vi "CRYSet Plot Settings.vi"(4 "Fill To":i16, 6 "Style":u8, 7 "sAction":string, 8 "Color":u32, 9 "Row":i32, 10 "Legend Refnum":refnum<vi>, 11 "Type":enum16{"Curves", "Values", "Results", "WFM"}(ring)) -> ()   [LabVIEW 2013]
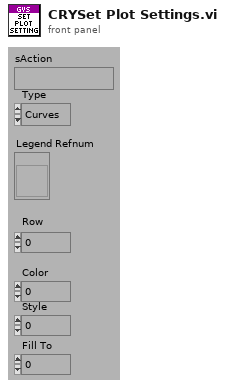
[diagram p1: front panel]
types:
  T1 = typedef "CRYData Cluster.ctl" = cluster{"Name":string, "Curve":cluster{"x":dbl, "y":dbl, "z":dbl}[], "X data":u16, "Y data":u16, "Z data":u16, "X axis":u16, "Y axis":u16, "Z axis":u16, "X unit":string, "Y unit":string, "Z unit":string, "X dB ref":dbl, "Y dB ref":dbl, "Z dB ref":dbl, "single val":bool, "protected":bool, "display X":bool, "display Y":bool, "display Z":bool, "Test Info":string, "Step No.":i32, "Plot Settings":cluster{"Color":u32, "Interpolation":u8, "Point Style":u8, "Line Style":u8, "Point Color":u32, "Line Width":u8, "Bar Plot Style":u8, "Fill To":i16}, "AutoProtect":bool}
  T2 = typedef "CRYWaveform Cluster.ctl" = cluster{"Waveform":cluster{"X0":dbl, "dX":dbl, "Y":sgl[]}, "X data":u16, "Y data":u16, "Y axis":u16, "X unit":string, "Y unit":string, "Y dB ref":dbl, "display Y":bool, "display X":bool, "Overload?":bool, "Test Info":string, "Step No.":i32, "Name":string, "protected":bool, "Sqc history":string[], "Signal Channel ID":i32, "Plot Settings":cluster{"Color":u32, "Interpolation":u8, "Point Style":u8, "Line Style":u8, "Point Color":u32, "Line Width":u8, "Bar Plot Style":u8, "Fill To":i16}, "AutoProtect":bool}
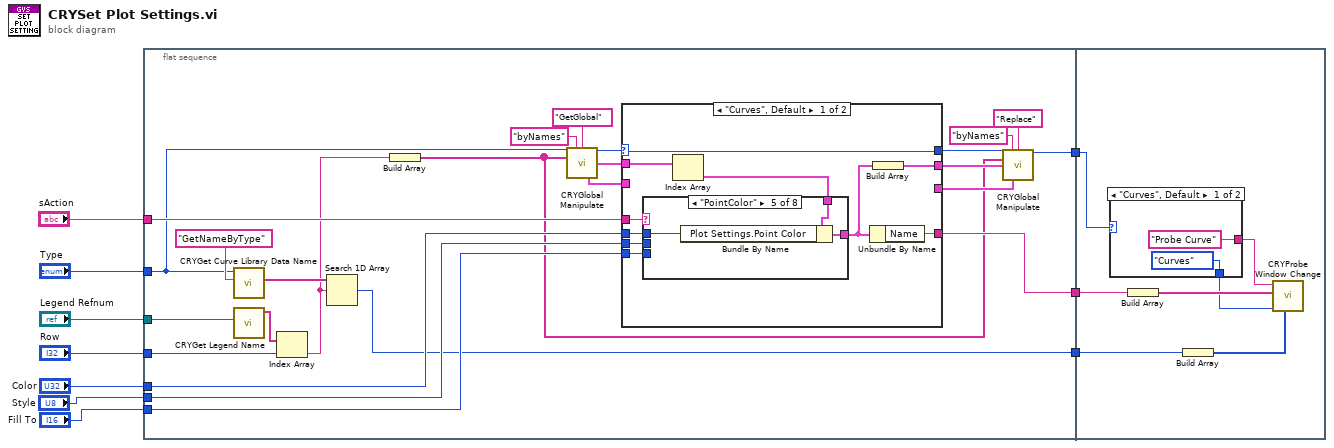
[diagram p0: block diagram]
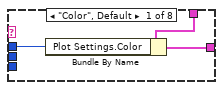
[diagram p2: hidden frame]
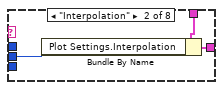
[diagram p3: hidden frame]
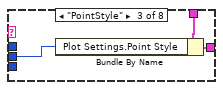
[diagram p4: hidden frame]
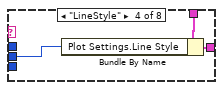
[diagram p5: hidden frame]
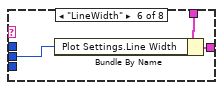
[diagram p6: hidden frame]
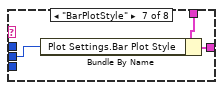
[diagram p7: hidden frame]
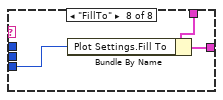
[diagram p8: hidden frame]
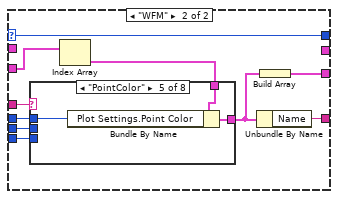
[diagram p9: hidden frame]
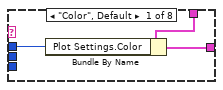
[diagram p10: hidden frame]
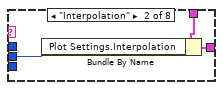
[diagram p11: hidden frame]
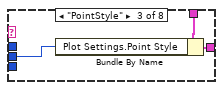
[diagram p12: hidden frame]
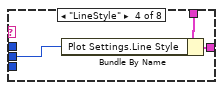
[diagram p13: hidden frame]
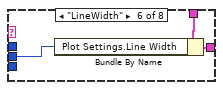
[diagram p14: hidden frame]
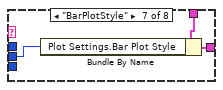
[diagram p15: hidden frame]
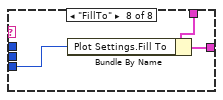
[diagram p16: hidden frame]
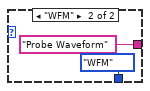
[diagram p17: hidden frame]
diagram:
  n1 = flat-sequence {
    tunnel: "Color" -> [w22]
    tunnel: "Legend Refnum" -> [w33]
    tunnel: "Row" -> [w32]
    tunnel: "Type" -> [w14]
    tunnel: [w18] -> w10
    tunnel: [w19] -> w9
    tunnel: "sAction" -> [w23]
    tunnel: "Style" -> [w21]
    tunnel: "Fill To" -> [w20]
    tunnel: [w17] -> w1
    tunnel: w10 -> [w109]
    tunnel: w9 -> [w106]
    tunnel: w1 -> [w104]
    frame #0 {
      n2 = call "CRYGet Curve Library Data Name.vi"("sAction"="GetNameByType", "Type"=w14) -> ("sNames"=w35:string[])  [unwired: 4 in, 5 out]
      n3 = call "CRYGet Legend Name.vi"("MCListbox Refnum"=w33) -> ("Names Out"=w34:string[])  [unwired: 1 in, 9 out]
      n4 = Index Array(array=w34, index=w32) -> (element=w13:string)
      n5 = Search 1D Array(1D array=w35, element=w13) -> (index of element=w19:i32)  [unwired: 1 in]
      n6 = Build Array(w13) -> (w12:string[])
      n7 = call "CRYGlobal Manipulate.vi"("Type"=w14, "sOption"="byNames", "sAction"="GetGlobal", "sData"=w12) -> ("Type out"=w16:enum16{"Curves", "Values", "Results", "WFM"}, "Curves Out"=w30:T1[], "WFM Out"=w25:T2[])  [unwired: 5 in, 4 out]
      n8 = case shown="\"Curves\", Default" w16 {
        selector: w16 -> [w36 w70]
        tunnel: w30 -> [w45 _]
        tunnel: [w37 _] -> w26
        tunnel: w25 -> [_ w72]
        tunnel: [_ w71] -> w24
        tunnel: [w43 w78] -> w18
        tunnel: w23 -> [w42 w77]
        tunnel: w22 -> [w41 w76]
        tunnel: w21 -> [w40 w75]
        tunnel: w20 -> [w39 w74]
        tunnel: [w36 w70] -> w15
        frame "Curves", Default {
          n9 = Index Array(array=w45) -> (element=w44:T1)  [unwired: 1 in]
          n10 = case shown="\"PointColor\"" w42 {
            tunnel: w41 -> [w48 _ _ _ w60 _ _ _]
            tunnel: w44 -> [w46 w51 w54 w57 w59 w63 w66 w69]
            tunnel: [w47 w50 w53 w56 w58 w62 w65 w68] -> w38
            tunnel: w40 -> [_ w49 w52 w55 _ w61 w64 _]
            tunnel: w39 -> [_ _ _ _ _ _ _ w67]
            frame "Color", Default {
              n11 = Bundle By Name(cluster=w46, "Plot Settings.Color"=w48) -> (w47:T1)
            }
            frame "Interpolation" {
              n12 = Bundle By Name(cluster=w51, "Plot Settings.Interpolation"=w49) -> (w50:T1)
            }
            frame "PointStyle" {
              n13 = Bundle By Name(cluster=w54, "Plot Settings.Point Style"=w52) -> (w53:T1)
            }
            frame "LineStyle" {
              n14 = Bundle By Name(cluster=w57, "Plot Settings.Line Style"=w55) -> (w56:T1)
            }
            frame "PointColor" {
              n15 = Bundle By Name(cluster=w59, "Plot Settings.Point Color"=w60) -> (w58:T1)
            }
            frame "LineWidth" {
              n16 = Bundle By Name(cluster=w63, "Plot Settings.Line Width"=w61) -> (w62:T1)
            }
            frame "BarPlotStyle" {
              n17 = Bundle By Name(cluster=w66, "Plot Settings.Bar Plot Style"=w64) -> (w65:T1)
            }
            frame "FillTo" {
              n18 = Bundle By Name(cluster=w69, "Plot Settings.Fill To"=w67) -> (w68:T1)
            }
          }
          n19 = Unbundle By Name(w38) -> ("Name"=w43:string)
          n20 = Build Array(w38) -> (w37:T1[])
        }
        frame "WFM" {
          n21 = Index Array(array=w72) -> (element=w79:T2)  [unwired: 1 in]
          n22 = case shown="\"PointColor\"" w77 {
            tunnel: w76 -> [w82 _ _ _ w94 _ _ _]
            tunnel: w79 -> [w80 w85 w88 w91 w93 w97 w100 w103]
            tunnel: [w81 w84 w87 w90 w92 w96 w99 w102] -> w73
            tunnel: w75 -> [_ w83 w86 w89 _ w95 w98 _]
            tunnel: w74 -> [_ _ _ _ _ _ _ w101]
            frame "Color", Default {
              n23 = Bundle By Name(cluster=w80, "Plot Settings.Color"=w82) -> (w81:T2)
            }
            frame "Interpolation" {
              n24 = Bundle By Name(cluster=w85, "Plot Settings.Interpolation"=w83) -> (w84:T2)
            }
            frame "PointStyle" {
              n25 = Bundle By Name(cluster=w88, "Plot Settings.Point Style"=w86) -> (w87:T2)
            }
            frame "LineStyle" {
              n26 = Bundle By Name(cluster=w91, "Plot Settings.Line Style"=w89) -> (w90:T2)
            }
            frame "PointColor" {
              n27 = Bundle By Name(cluster=w93, "Plot Settings.Point Color"=w94) -> (w92:T2)
            }
            frame "LineWidth" {
              n28 = Bundle By Name(cluster=w97, "Plot Settings.Line Width"=w95) -> (w96:T2)
            }
            frame "BarPlotStyle" {
              n29 = Bundle By Name(cluster=w100, "Plot Settings.Bar Plot Style"=w98) -> (w99:T2)
            }
            frame "FillTo" {
              n30 = Bundle By Name(cluster=w103, "Plot Settings.Fill To"=w101) -> (w102:T2)
            }
          }
          n31 = Unbundle By Name(w73) -> ("Name"=w78:string)
          n32 = Build Array(w73) -> (w71:T2[])
        }
      }
      n33 = call "CRYGlobal Manipulate.vi"("Type"=w15, "sOption"="byNames", "sAction"="Replace", "sData"=w12, "Curves"=w26, "WFM"=w24) -> ("Type out"=w17:enum16{"Curves", "Values", "Results", "WFM"})  [unwired: 3 in, 6 out]
    }
    frame #1 {
      n34 = case shown="\"Curves\", Default" w104 {
        tunnel: ["Probe Curve" "Probe Waveform"] -> w110
        tunnel: [enum16{"Curves", "Values", "Results", "WFM"}."Curves" ("Type") enum16{"Curves", "Values", "Results", "WFM"}."WFM" ("Type")] -> w107
        frame "Curves", Default {
        }
        frame "WFM" {
        }
      }
      n35 = Build Array(w109) -> (w108:string[])
      n36 = Build Array(w106) -> (w105:i32[])
      n37 = call "CRYProbe Window Change.vi"("Update Index"=w105, "Type"=w107, "Update Names"=w108, "Probe Type"=w110) -> ()  [unwired: 1 in, 7 out]
    }
  }
